vi "Write FIU.vi"(8 "error in (no error)":errorcluster, 10 "FIU Engine Refs in":T1 {"FIU IDs"."Slot #" max=15; "FIU IDs"."Chip Address (A2 A1 A0)" max=7; "FIU Block Data Refs"."Data Reference" format="%.0x"}, 11 "DMA FIFO Ref in":refnum<k20>) -> (0 "error out":errorcluster, 2 "FIU Engine Refs out":T1 {"FIU IDs"."Slot #" max=15; "FIU IDs"."Chip Address (A2 A1 A0)" max=7; "FIU Block Data Refs"."Data Reference" format="%.0x"}, 3 "DMA FIFO Ref out":refnum<k20>)   [LabVIEW 2014, in "SLSC configuration Engine.lvlib"]
uses:
  SLSC configuration Engine.lvlib
  Type Defs/FIU Engine Refs.ctl
  Shared/Type Defs/FIU IDs.ctl
  Example/SPI Utility/Slot #.ctl
  Example/MCP23S17/Chip Address.ctl
  <vilib>/NI Veristand/Custom Device API/Block Data Reference.ctl
  <vilib>/NI Veristand/Custom Device API/Data Reference.ctl
  <vilib>/NI Veristand/Custom Device API/Global Data Refs.vi
  <vilib>/Utility/error.llb/Error Cluster From Error Code.vi
  <vilib>/rvi/errors/niLvFpgaAdjustHostInterfaceError.vi
  <vilib>/rvi/interface/nirviMethod/nirviMethod.xnode
  <vilib>/NI Veristand/Custom Device API/Custom Device API.lvlib
  Shared/SLSC configuration Shared.lvlib
  <vilib>/FPGAPlugInAG/Dynamic/niLvFpga_WriteFifo_Dynamic.vi
  <vilib>/rvi/errors/niLvFpgaMergeErrorWithErrorCode.vi
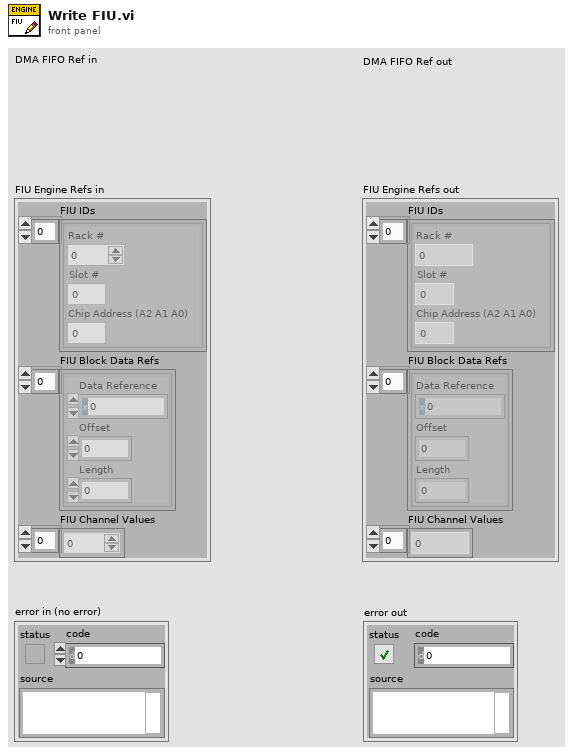
[diagram p1: front panel]
types:
  T1 = typedef "SLSC configuration Engine.lvlib/FIU Engine Refs.ctl" = cluster{"FIU IDs":T2[], "FIU Block Data Refs":T5[], "FIU Channel Values":dbl[]}
  T2 = typedef "SLSC configuration Shared.lvlib/FIU IDs.ctl" = cluster{"Rack #":u8, "Slot #":T3, "Chip Address (A2 A1 A0)":T4}
  T3 = typedef "SLSC configuration Shared.lvlib/Slot #.ctl" = u8
  T4 = typedef "SLSC configuration Shared.lvlib/Chip Address.ctl" = u8
  T5 = typedef "Custom Device API.lvlib/Block Data Reference.ctl" = cluster{"Data Reference":T6, "Offset":i32, "Length":i32}
  T6 = typedef "Custom Device API.lvlib/Data Reference.ctl" = i32
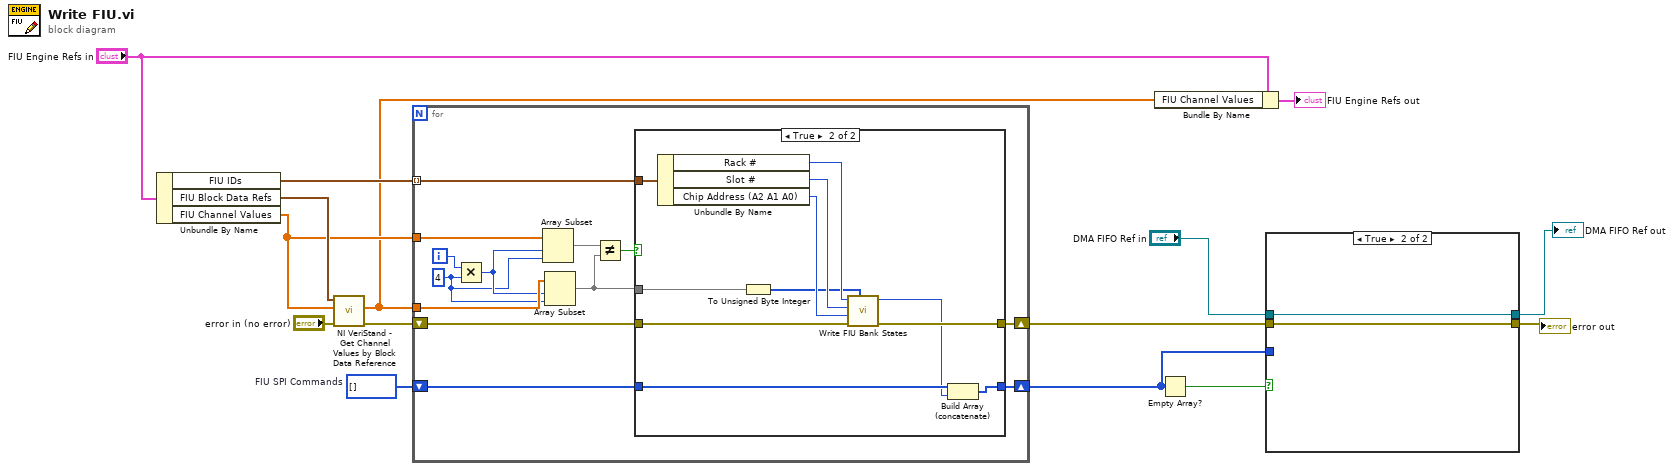
[diagram p0: block diagram]
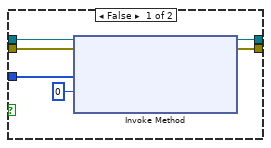
[diagram p2: hidden frame]
diagram:
  w7 = u64[] []  # FIU SPI Commands
  n1 = Unbundle By Name("FIU Engine Refs in") -> ("FIU IDs"=w12:T2[], "FIU Block Data Refs"=w15:T5[], "FIU Channel Values"=w10:dbl[])
  n2 = call <vilib>:"NI VeriStand - Get Channel Values by Block Data Reference.vi"("error in (no error)"="error in (no error)", "Values Array in"=w10, "Block Data Ref"=w15) -> ("error out"=w13:errorcluster, "Values Array out"=w9:dbl[])  [unwired: 6 in, 1 out]
  n3 = for {
    shift-right: [w19] -> w6
    shift-left: w13 -> [w21]
    tunnel: w12 -> [w22] mode=indexing
    tunnel: w9 -> [w26]
    tunnel: w10 -> [w27]
    shift-right: [w16] -> w3
    shift-left: w7 -> [w17]
    i -> [w28]
    w24 = 4 ("y")
    n4 = Multiply(x=w28, y=w24) -> (x*y=w25:i32)
    n5 = Array Subset(array=w27, index=w25, length=w24) -> (w23:dbl[])
    n6 = Array Subset(array=w26, index=w25, length=w24) -> (w20:dbl[])
    n7 = Not Equal?(x=w23, y=w20) -> (x != y?=w18:bool)
    n8 = case shown="True" w18 {
      tunnel: w22 -> [_ w41]
      tunnel: w21 -> [w30 w40]
      tunnel: w20 -> [_ w36]
      tunnel: [w30 w34] -> w19
      tunnel: w17 -> [w29 w33]
      tunnel: [w29 w31] -> w16
      frame False {
      }
      frame True {
        n9 = Unbundle By Name(w41) -> ("Rack #"=w39:u8, "Slot #"=w38:T3, "Chip Address (A2 A1 A0)"=w37:T4)
        n10 = To Unsigned Byte Integer(number=w36) -> (unsigned 8bit integer=w35:u8[])
        n11 = call "Write FIU Bank States.vi"("Fault States"=w35, "error in (no error)"=w40, "Chip Address (A2 A1 A0)"=w37, "Slot #"=w38, "Rack #"=w39) -> ("error out"=w34:errorcluster, "FIFO SPI Message"=w32:u64)  [unwired: 4 in, 1 out]
        n12 = Build Array (concatenate)(w33, w32) -> (w31:u64[])
      }
    }
  }
  n13 = Bundle By Name(cluster="FIU Engine Refs in", "FIU Channel Values"=w9) -> (→"FIU Engine Refs out":T1)
  n14 = Empty Array?(array=w3) -> (empty?=w5:bool)
  n15 = case shown="True" w5 {
    tunnel: "DMA FIFO Ref in" -> [w47 w48]
    tunnel: w6 -> [w45 w49]
    tunnel: [w44 w49] -> w4
    tunnel: w3 -> [w43 _]
    tunnel: [w42 w48] -> w1
    frame False {
      n16 = xnode "Invoke Method"("FPGA VI Reference In"=w47, "error in"=w45, "Data"=w43, "Timeout (ms)"=0) -> ("FPGA VI Reference Out"=w42:refnum<k20>, "error out"=w44:errorcluster)  [unwired: 1 out]
    }
    frame True {
    }
  }
  "error out" <- w4
  "DMA FIFO Ref out" <- w1
